vi "Close.vi"(8 "error in (no error)":errorcluster, 11 "Pump_1AI_1DO_2DI in":refnum<class "Valve_2DO_2DI.lvclass">) -> (0 "error out":errorcluster, 3 "Pump_1AI_1DO_2DI out":refnum<class "Valve_2DO_2DI.lvclass">)   [LabVIEW 2019, in "Valve_2DO_2DI.lvclass"]
uses:
  Valve_2DO_2DI.lvclass
  Valve_2DO_2DI.lvclass/Valve_2DO_2DI.ctl
  FPGA/TypeDef/valveState.ctl
  FPGA_API_class/FPGA API.lvclass
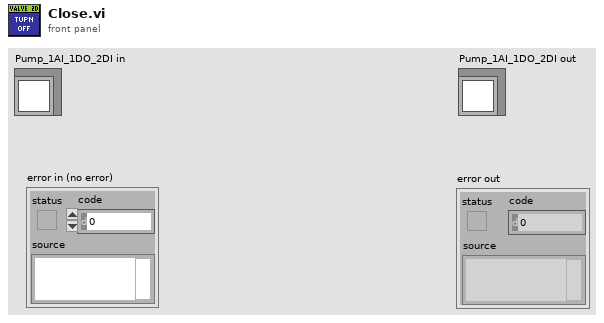
[diagram p1: front panel]
types:
  T1 = typedef "valveState.ctl" = enum16{"Closed", "Opening", "Opened", "Closing"}
  T2 = typedef "DO index.ctl" = u8
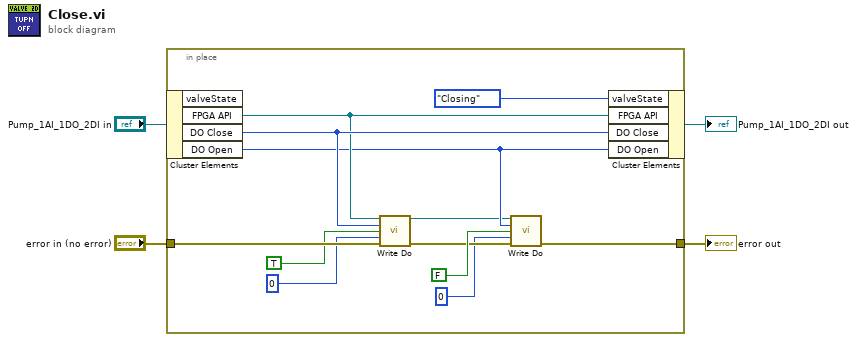
[diagram p0: block diagram]
diagram:
  n1 = in-place {
    in-place-border: "error in (no error)" -> [w15]
    in-place-border: [w13] -> w1
    n2 = in-place-cluster #1("Pump_1AI_1DO_2DI in") -> ("FPGA API"=w14:refnum<class "FPGA API.lvclass">, "DO Close"=w16:T2, "DO Open"=w12:T2)  [unwired: 1 out]
    n3 = call "Write Do.vi"("FPGA API in"=w14, "#DO"=w16, "value"=TRUE, "Time uSec"=u32 0, "error in (no error)"=w15) -> ("FPGA API out"=w6:refnum<class "FPGA API.lvclass">, "error out"=w7:errorcluster)  [unwired: 9 in]
    n4 = call "Write Do.vi"("FPGA API in"=w6, "#DO"=w12, "value"=FALSE, "Time uSec"=u32 0, "error in (no error)"=w7) -> ("error out"=w13:errorcluster)  [unwired: 9 in, 1 out]
    n5 = in-place-cluster #1("valveState"=valveState."Closing", "FPGA API"=w14, "DO Close"=w16, "DO Open"=w12) -> (→"Pump_1AI_1DO_2DI out":refnum<class "Valve_2DO_2DI.lvclass">)
  }
  "error out" <- w1
